vi "StMotor_dir.vi"() -> ()   [LabVIEW 2018]
doc: "This example shows how to use the Arduino Stepper Motor API. The fritzing diagram shows use with the EasyStepper 4.3 or 4.4 motor controller."
uses:
  <vilib>/LabVIEW Interface for Arduino/Type Defs/Connection Type.ctl
  <vilib>/LabVIEW Interface for Arduino/Type Defs/Board Type.ctl
  <vilib>/LabVIEW Interface for Arduino/LabVIEW Interface for Arduino.lvlib
panel:
  in  "Set Speed":i16=100
  out "NewVal":i16
  out "OldVal":i16
  in  "Board Type (Uno)":T1
  in  "Connection Type (USB/Serial)":T2
  in  "Baud Rate (9600)":u32=115200
  in  "VISA resource":refnum<visa-resource-name>
  in  "Stop":bool
  in  "Stepper #":u8=1
  in  "OK Button":bool
  in  "Set Acceleration (0 to disable)":i16
  in  "# of Steps to Move":i16
  in  "Set Speed (Steps per Second)":i16=100
  out "Steps Remaining?":bool
  in  "Dial":i16(knob) scale=0.0..200.0
  in  "error in":errorcluster
  # "Preset Movement"
  # "Interactive Movement"
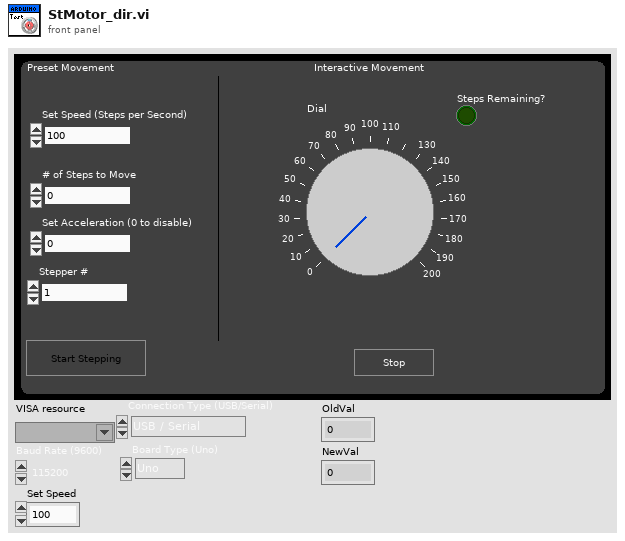
[diagram p1: front panel]
types:
  T1 = typedef "LabVIEW Interface for Arduino.lvlib/Board Type.ctl" = enum16{"Uno", "Dimuelanove w/Atmega 328", "Mega 2560"}
  T2 = typedef "LabVIEW Interface for Arduino.lvlib/Connection Type.ctl" = enum8{"USB / Serial", "XBEE", "BlueSmirf (Bluetooth)"}
  T3 = typedef "LabVIEW Interface for Arduino.lvlib/Arduino Resource.ctl" = cluster{"VISA resource":refnum<visa-resource-name>, "Board Type":T1, "Connection Type":enum8{"USB / Serial"}, "Bytes Per Packet (15)":u8}
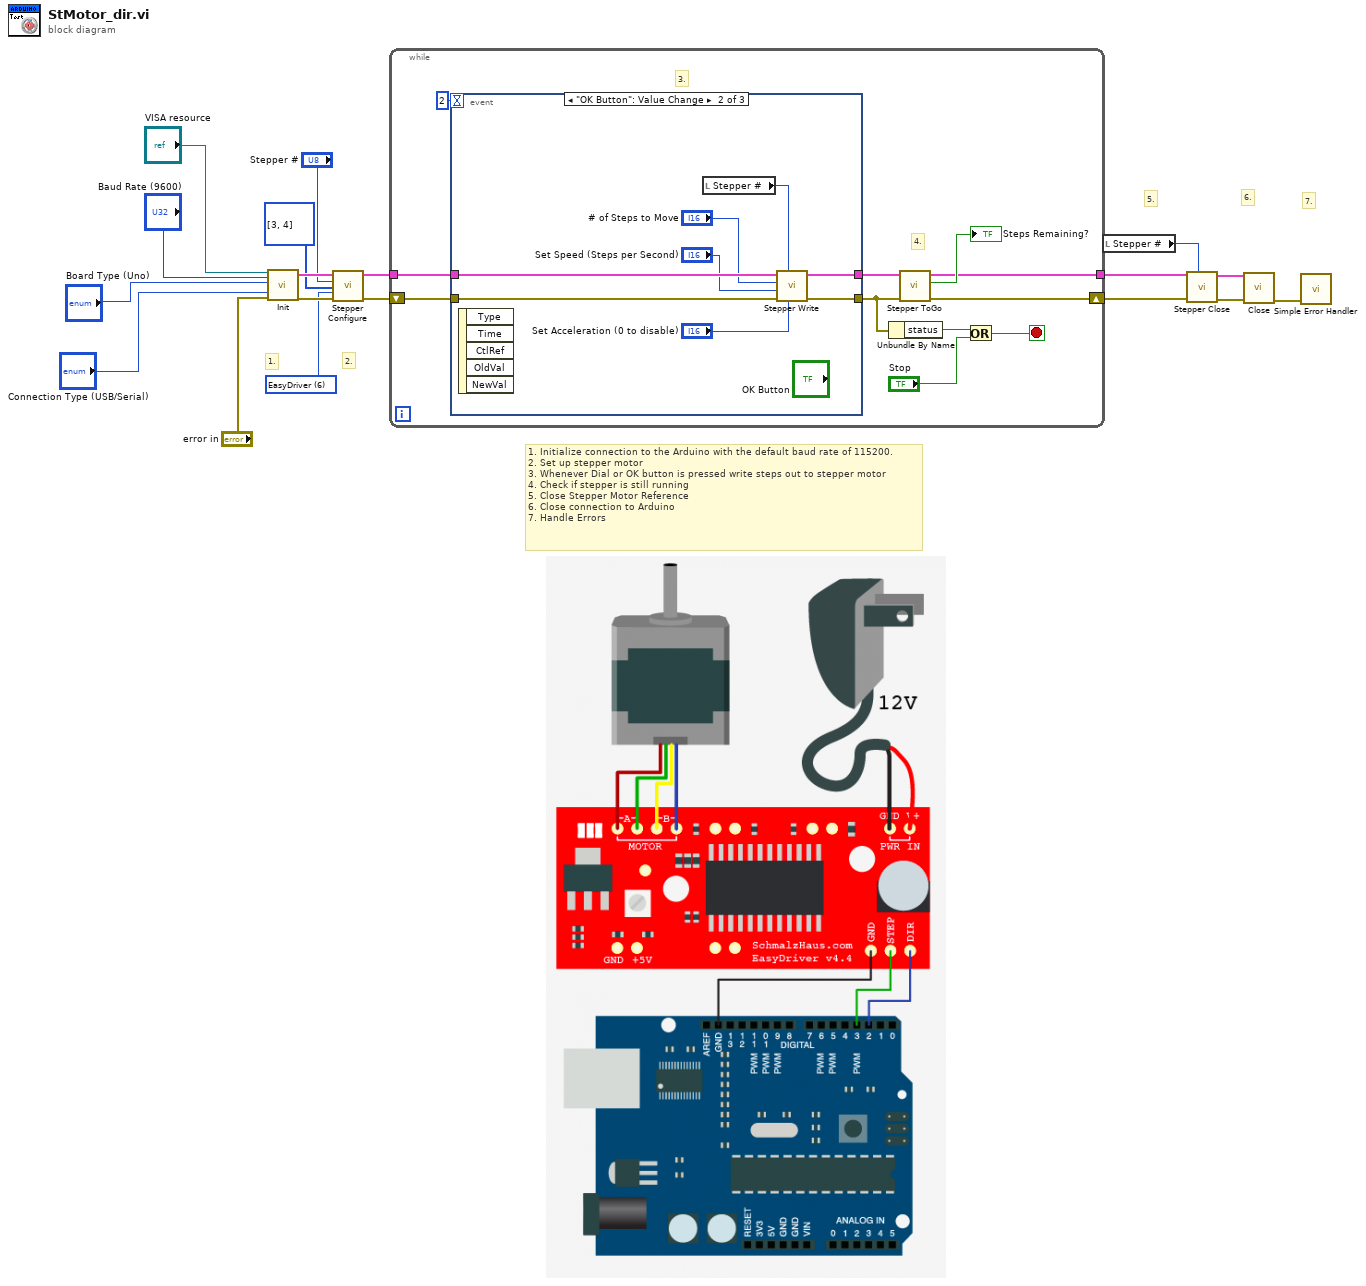
[diagram p0: block diagram]
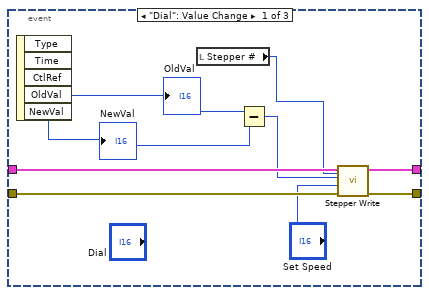
[diagram p2: hidden frame]
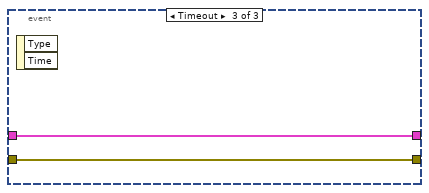
[diagram p3: hidden frame]
diagram:
  w6 = u8 6 items=["2 Wire (Pulse & Direction)"=1, "2 Wire"=2, "4 Wire"=4, "EasyDriver"=6, "AF Motor Shield (Stepper 1 & 2 Only)"=5] ("Control Method")
  # "7."
  # "6."
  # "5."
  # "2."
  # "1."
  # "1. Initialize connection to the Arduino with the default baud rate of 115200.\n2. Set up stepper motor\n3. Whenever Dial or OK button is pressed write steps out to stepper motor\n4. Check if stepper is still running\n5. Close Stepper Motor Reference \n6. Close connection to Arduino\n7. Handle Errors"
  n1 = call <vilib>:"Init.vi"("VISA resource"="VISA resource", "Baud Rate (115200)"="Baud Rate (9600)", "Board Type (Uno)"="Board Type (Uno)", "Connection Type (USB/Serial)"="Connection Type (USB/Serial)", "error in"="error in") -> ("Arduino Resource"=w9:T3, "error out"=w8:errorcluster)  [unwired: 13 in]
  n2 = call <vilib>:"Stepper Configure.vi"("Control Method"=w6, "Stepper #"="Stepper #", "error in"=w8, "Stepper Pins"=u8[] [3, 4], "Arduino Resource"=w9) -> ("error out"=w16:errorcluster, "Arduino Resource Out"=w17:T3)  [unwired: 5 in]
  n3 = while {
    tunnel: w17 -> [w28]
    tunnel: [w22] -> w15
    shift-right: [w20] -> w14
    shift-left: w16 -> [w29]
    stop <- w26 stop-if-true
    # "4."
    # "3."
    n4 = event shown="[1] \"OK Button\": Value Change" {
      selector: _ -> [_ _ _]
      dyn-events: _ -> [_ _ _]
      timeout: 2 -> [_ _ _]
      tunnel: w29 -> [w38 w45 w47]
      tunnel: w28 -> [w37 w43 w48]
      tunnel: [w36 w44 w48] -> w24
      tunnel: [w35 w46 w47] -> w21
      event "Dial": Value Change {
        n5 = event-data() -> ("OldVal"=w30:i16, "NewVal"=w31:i16)  [unwired: 1 in, 3 out]
        "OldVal" <- w30
        "NewVal" <- w31
        n6 = local read "Stepper #"() -> (w33:u8)
        n7 = Subtract(x=w30, y=w31) -> (x-y=w32:i16)
        n8 = call <vilib>:"Stepper Write.vi"("Stepper #"=w33, "error in"=w38, "Set Speed (Steps per Second)"="Set Speed", "# of Steps to Move"=w32, "Arduino Resource"=w37) -> ("error out"=w35:errorcluster, "Arduino Resource Out"=w36:T3)  [unwired: 5 in]
      }
      event "OK Button": Value Change {
        n9 = event-data() -> ()  [unwired: 1 in, 5 out]
        n10 = local read "Stepper #"() -> (w39:u8)
        n11 = call <vilib>:"Stepper Write.vi"("Set Acceleration (0 to disable)"="Set Acceleration (0 to disable)", "Stepper #"=w39, "error in"=w45, "Set Speed (Steps per Second)"="Set Speed (Steps per Second)", "# of Steps to Move"="# of Steps to Move", "Arduino Resource"=w43) -> ("error out"=w46:errorcluster, "Arduino Resource Out"=w44:T3)  [unwired: 4 in]
      }
      event Timeout {
        n12 = event-data() -> ()  [unwired: 1 in, 2 out]
      }
    }
    n13 = Unbundle By Name(w21) -> ("status"=w25:bool)
    n14 = call <vilib>:"Stepper ToGo.vi"("error in"=w21, "Arduino Resource"=w24) -> ("error out"=w20:errorcluster, "Steps Remaining?"=→"Steps Remaining?":bool, "Arduino Resource Out"=w22:T3)  [unwired: 6 in, 1 out]
    n15 = Or(x=w25, y="Stop") -> (x .or. y?=w26:bool)
  }
  n16 = local read "Stepper #"() -> (w10:u8)
  n17 = call <vilib>:"Stepper Close.vi"("Stepper #"=w10, "error in"=w14, "Arduino Resource"=w15) -> ("error out"=w13:errorcluster, "Arduino Resource Out"=w12:T3)  [unwired: 7 in]
  n18 = call <vilib>:"Close.vi"("Arduino Resource"=w12, "error in"=w13) -> ("error out"=w18:errorcluster)  [unwired: 13 in]
  n19 = call <vilib>:"Simple Error Handler.vi"("error in (no error)"=w18) -> ()  [unwired: 4 in, 5 out]
